vi "XML-String in Typen-Array.vi"(1 "XML-String":string) -> (0 "Typen (ohne Cluster)":string[](array[string]))   [LabVIEW 2020, in "Anlagenuebersicht.lvlib" / "VisBx Anzeige.lvlib"]
uses:
  VisBx Anzeige.lvlib
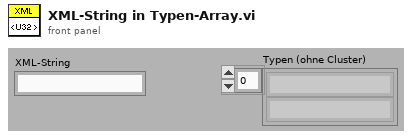
[diagram p1: front panel]
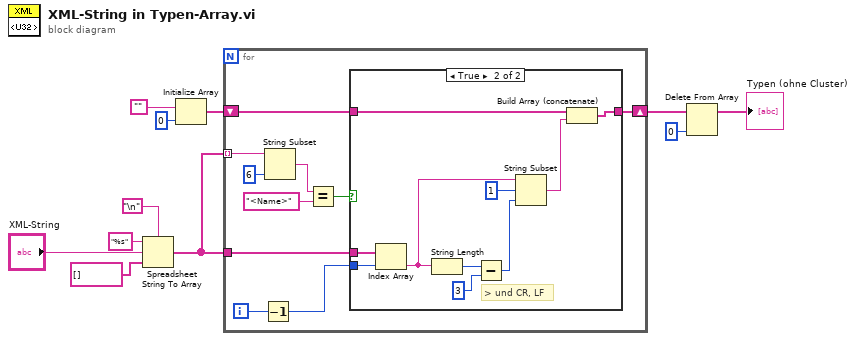
[diagram p0: block diagram]
diagram:
  n1 = Spreadsheet String To Array(delimiter (Tab)="\n", format string="%s" ("Format-String"), spreadsheet string="XML-String", array type (2D Dbl)=string[] []) -> (array=w5:string[])
  n2 = Initialize Array("", 0 ("Dimension")) -> (w4:string[])
  n3 = for {
    tunnel: w5 -> [w21] mode=indexing
    tunnel: w5 -> [w16]
    shift-right: [w12] -> w1
    shift-left: w4 -> [w13]
    i -> [w15]
    n4 = Decrement(x=w15) -> (x-1=w14:i32)
    n5 = String Subset(string=w21, length (rest)=6 ("Länge (Rest)")) -> (substring=w19:string)  [unwired: 1 out]
    n6 = Equal?(x=w19, y="<Name>") -> (x = y?=w17:bool)
    n7 = case shown="True" w17 {
      tunnel: w16 -> [_ w32]
      tunnel: w14 -> [_ w31]
      tunnel: w13 -> [w22 w30]
      tunnel: [w22 w23] -> w12
      frame False {
      }
      frame True {
        # "> und CR, LF"
        n8 = Index Array(array=w32, index=w31) -> (element=w28:string)
        n9 = String Length(string=w28) -> (length=w27:i32)
        n10 = Subtract(x=w27, y=3) -> (x-y=w25:i32)
        n11 = String Subset(string=w28, offset (0)=1 ("Offset (0)"), length (rest)=w25) -> (substring=w24:string)
        n12 = Build Array (concatenate)(w30, w24) -> (w23:string[])
      }
    }
  }
  n13 = Delete From Array(array=w1, index=0 ("Index")) -> (array with subset deleted=→"Typen (ohne Cluster)":string[])  [unwired: 1 in, 1 out]
